vi "Database-SQLiteGetActiveConn.vi"(7 "PageID":string, 8 "error in (no error)":errorcluster, 11 "Database-Actor in":refnum<class "Database-Actor.lvclass">) -> (0 "error out":errorcluster, 2 "Active Plugin Caller":refnum<class "FTW-ActorConnector.lvclass">, 3 "Database-Actor out":refnum<class "Database-Actor.lvclass">)   [LabVIEW 2013, in "Database-Actor.lvclass"]
uses:
  Database-Actor.lvclass
  ftw-dataflow/Actor/src/Connector/FTW-ActorConnector.lvclass
  Database-Actor.lvclass/Database-Actor.ctl
  ftw-dataflow/Actor/src/Utility/FTW-Actor-Configuration.ctl
  ftw-dataflow/Core/src/Time/FTW-Time-Uptime.vi
  ftw-dataflow/Core/src/Database/FTW-SQLite-PrepareStatement.vi
  ftw-dataflow/Core/src/Database/FTW-SQLite-LibraryFilepath.vi
  ftw-dataflow/Core/src/Database/FTW-SQLite-LibraryReturnValue.vi
  ftw-dataflow/Core/src/Error/FTW-ERR-StatusOK.vi
  ftw-dataflow/Core/src/Error/FTW-ERR-ThrowImpossibleError.vi
  ftw-dataflow/Core/utils/CodeGen/SQLite-Fetch/FTW-SQLite-Fetch.xnode
  ftw-dataflow/Core/src/Database/FTW-SQLite-Connector.lvclass
  ftw-dataflow/Actor/src/FTW-Actor.lvlib
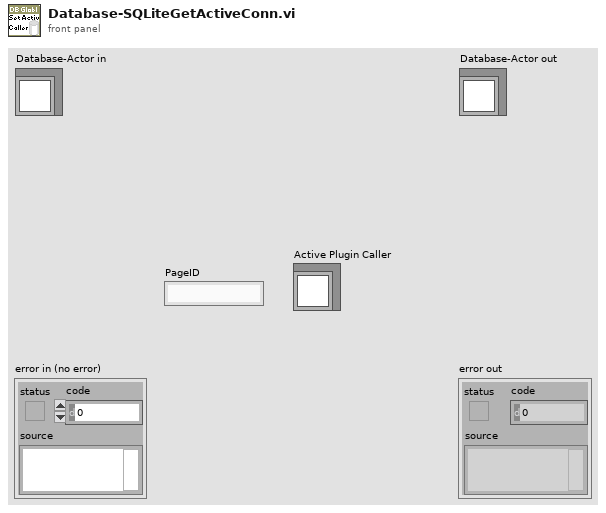
[diagram p1: front panel]
types:
  T1 = typedef "FTW-Actor.lvlib/FTW-Actor-Configuration.ctl" = string
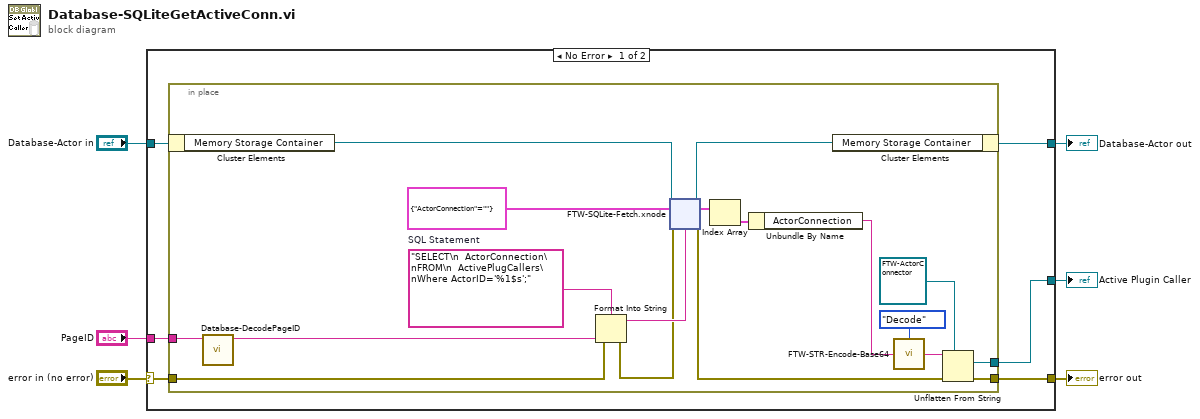
[diagram p0: block diagram]
diagram:
  n1 = case shown="No Error" "error in (no error)" {
    selector: "error in (no error)" -> [w8 w144]
    tunnel: [w7 w144] -> w5
    tunnel: [w10 w143] -> w3
    tunnel: "Database-Actor in" -> [w11 w143]
    tunnel: [w12 _] -> w2
    tunnel: "PageID" -> [w9 _]
    frame No Error {
      n2 = in-place {
        in-place-border: w8 -> [w20]
        in-place-border: [w19] -> w7
        in-place-border: w9 -> [w14]
        in-place-border: [w15] -> w12
        w29 = "SELECT\n  ActorConnection\nFROM\n  ActivePlugCallers\nWhere ActorID='%1$s';"  # SQL Statement
        n3 = in-place-cluster #1(w11) -> ("Memory Storage Container"=w30:refnum<class "FTW-SQLite-Connector.lvclass">)
        n4 = call "Database-DecodePageID.vi"("PageID"=w14) -> ("Decoded Page ID"=w13:string)  [unwired: 10 in]
        n5 = Format Into String(format string=w29, error in=w20, w13) -> (resulting string=w28:string, error out=w18:errorcluster)  [unwired: 1 in]
        n6 = xnode "FTW-SQLite-Fetch.xnode"("SQLite Connector"=w30, "SQL Script"=w28, "Row Datatype"=cluster{"ActorConnection":T1} {"ActorConnection"=""}, "error in"=w18) -> ("SQLite Connector out"=w27:refnum<class "FTW-SQLite-Connector.lvclass">, "Result Set"=w24:cluster{"ActorConnection":T1}[], "error out"=w17:errorcluster)  [unwired: 2 out]
        n7 = Index Array(array=w24) -> (element=w23:cluster{"ActorConnection":T1})  [unwired: 1 in]
        n8 = Unbundle By Name(w23) -> ("ActorConnection"=w22:T1)
        n9 = in-place-cluster #1("Memory Storage Container"=w27) -> (w10:refnum<class "Database-Actor.lvclass">)
        n10 = call "FTW-STR-Encode-Base64.vi"("Input"=w22, "Direction"=enum16{"Encode", "Decode"}."Decode") -> ("Output"=w21:string)
        n11 = Unflatten From String(type=refnum<class "FTW-ActorConnector.lvclass"> refnum ("Plugin Caller"), binary string=w21, error in (no error)=w17) -> (value=w15:refnum<class "FTW-ActorConnector.lvclass">, error out=w19:errorcluster)  [unwired: 2 in, 1 out]
      }
    }
    frame Error {
    }
  }
  "error out" <- w5
  "Database-Actor out" <- w3
  "Active Plugin Caller" <- w2
